vi "HMI_script_Generator.vi"(9 "Table Name":string, 10 "Columns":string[](array[string]), 11 "column information":T2(array[cluster])) -> (3 "HMI Script":string)   [LabVIEW 2020]
uses:
  <vilib>/addons/database/Auxilliary.llb/DB Tools DataTypes.ctl
  <userlib>/_OpenG.lib/array/array.llb/Search 1D Array (String)__ogtk.vi
  <userlib>/_OpenG.lib/array/array.llb/Delete Elements from 1D Array (String)__ogtk.vi
  <vilib>/regexp/Match Regular Expression.xnode
  <vilib>/addons/database/NI_Database_API.lvlib
panel:
  out "MACHINE NO":string
  out "Indices of Elements":i32[](array[numeric])
  out "column information 2":T2(array[cluster])
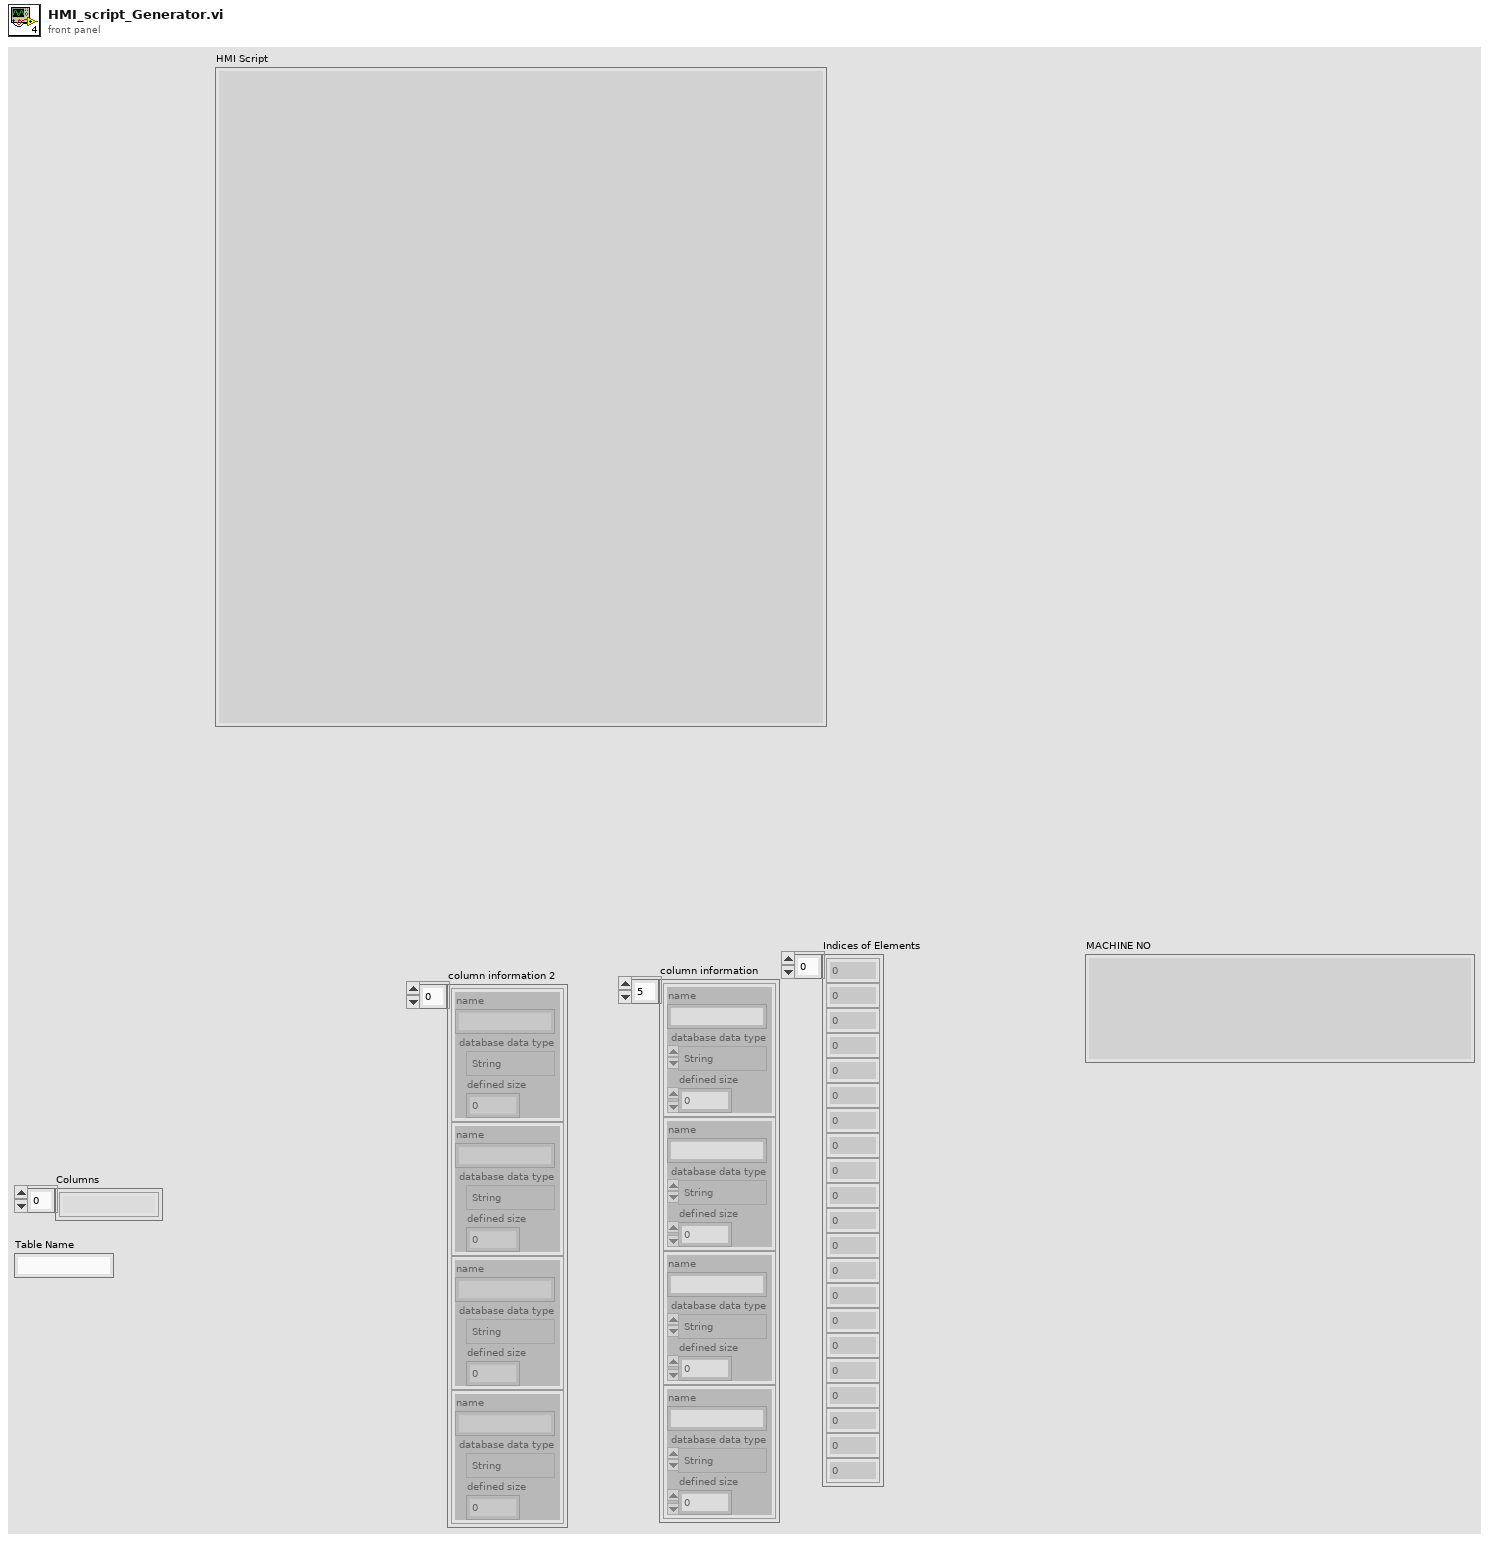
[diagram p1: front panel]
types:
  T1 = typedef "NI_Database_API.lvlib/DB Tools DataTypes.ctl" = enum16{"String", "Long (I32)", "Single (SGL)", "Double (DBL)", "Date/Time", "Binary"}
  T2 = cluster{"name":string, "database data type":T1, "defined size":i32}[]
  T3 = cluster{"name":string, "database data type":T1, "defined size":i32}
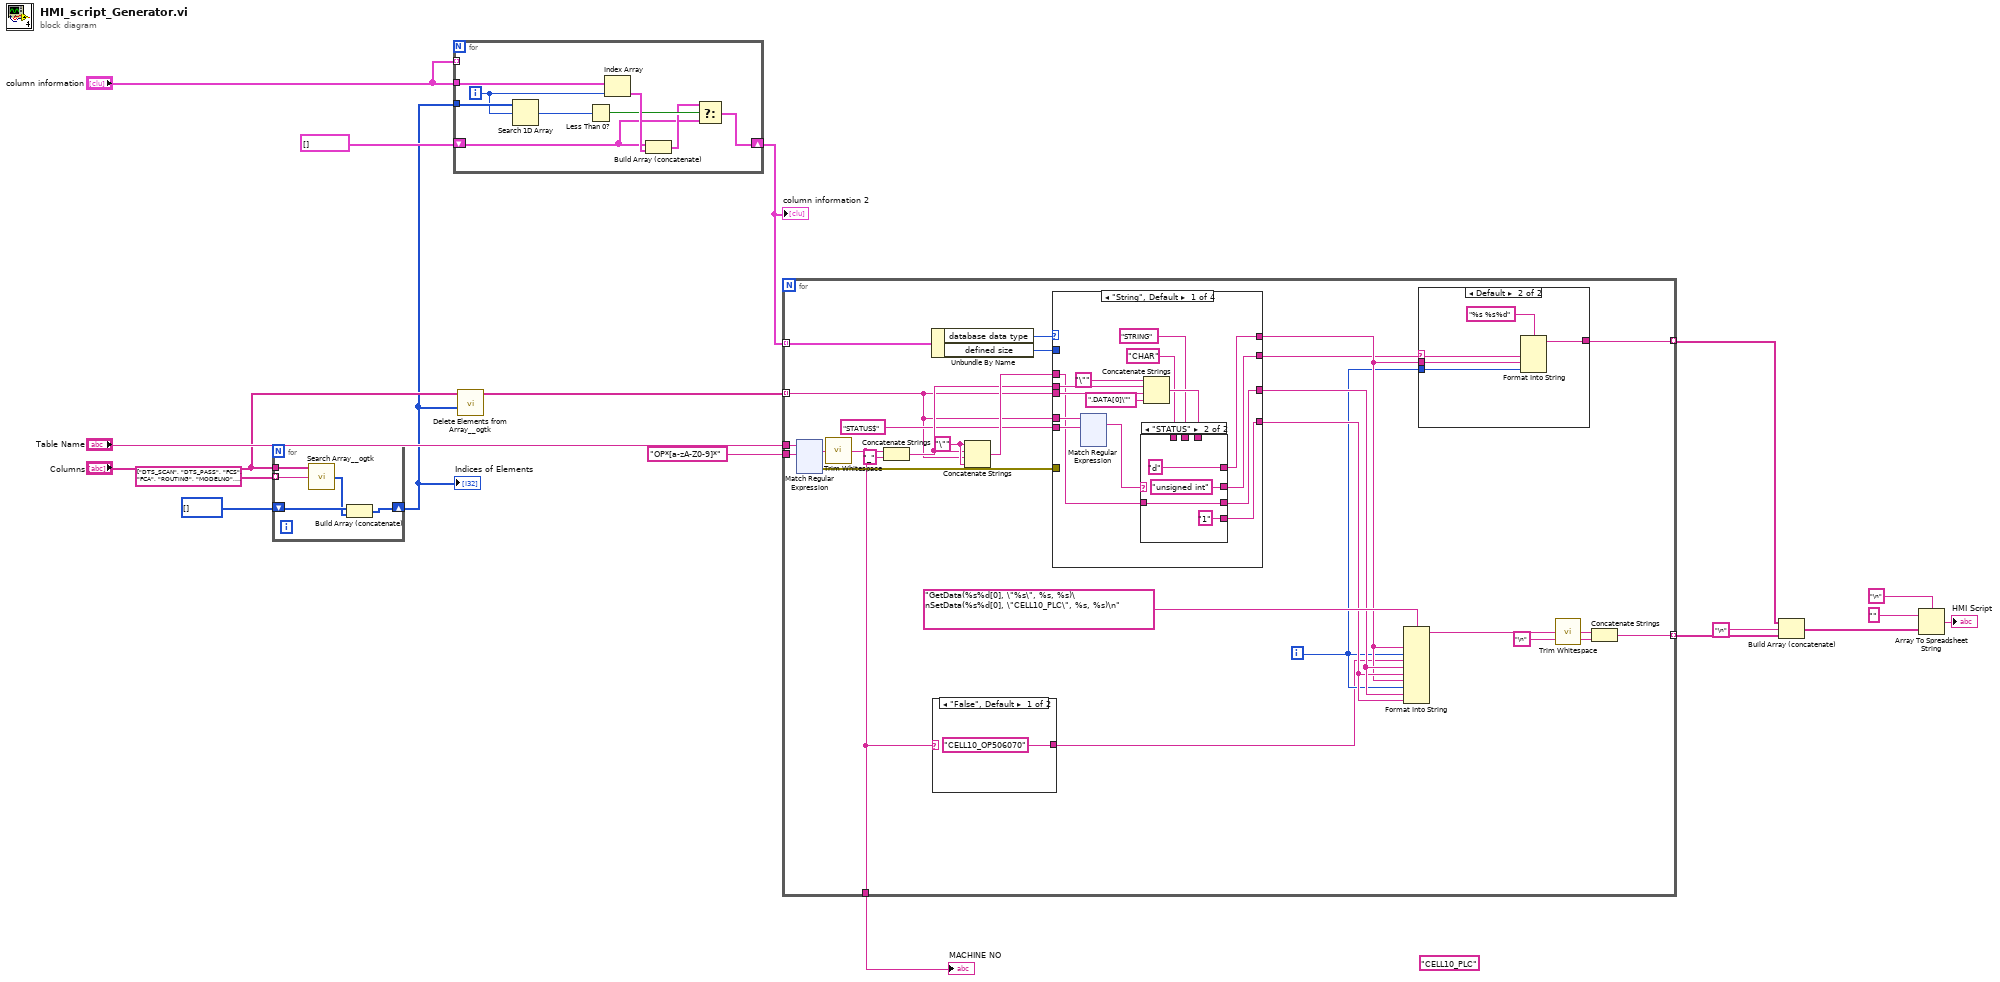
[diagram p0: block diagram]
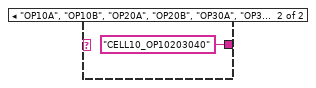
[diagram p2: hidden frame]
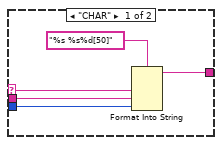
[diagram p3: hidden frame]
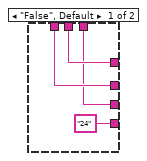
[diagram p4: hidden frame]
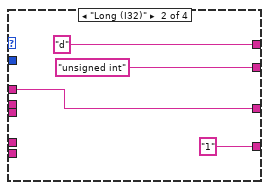
[diagram p5: hidden frame]
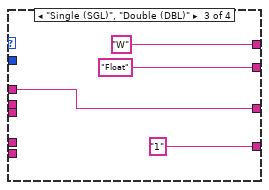
[diagram p6: hidden frame]
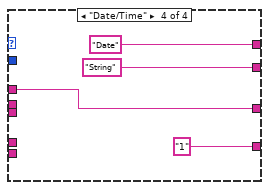
[diagram p7: hidden frame]
diagram:
  (unwired) "CELL10_PLC" ("format string")
  n1 = for {
    tunnel: "Columns" -> [w23]
    tunnel: string[] ["DTS_SCAN", "DTS_PASS", "FCS", "FCA", "ROUTING", "MODELNO", "WORKORDER", "CELLNO", "PROFITCENTRE", "MACHINECODE", "OPERATIONCODE"] ("columns") -> [w22] mode=indexing
    shift-right: [w20] -> w10
    shift-left: i32[] [] ("Indices of Elements") -> [w21]
    n2 = call-poly <userlib>:"Search Array__ogtk.vi"("Array"=w23, "Element Data"=w22) -> ("Indices of Elements"=w19:i32[])  [unwired: 7 in]
    n3 = Build Array (concatenate)(w21, w19) -> (w20:i32[])
  }
  "Indices of Elements" <- w10
  n4 = for {
    tunnel: "column information" -> [w32]
    shift-right: [w27] -> w14
    shift-left: T2 [] ("column information") -> [w28]
    tunnel: w10 -> [w26]
    tunnel: "column information" -> [_] mode=indexing
    i -> [w25]
    n5 = Search 1D Array(1D array=w26, element=w25) -> (index of element=w24:i32)  [unwired: 1 in]
    n6 = Less Than 0?(x=w24) -> (x < 0?=w30:bool)
    n7 = Index Array(array=w32, index=w25) -> (element=w31:T3)
    n8 = Build Array (concatenate)(w28, w31) -> (w29:T2)
    n9 = Select(t=w29, s=w30, f=w28) -> (s? t:f=w27:T2)
  }
  "column information 2" <- w14
  n10 = call-poly <userlib>:"Delete Elements from Array__ogtk.vi"("indices"=w10, "array"="Columns") -> ("array w/ subset deleted"=w12:string[])  [unwired: 8 in, 1 out]
  n11 = for {
    tunnel: w14 -> [w58] mode=indexing
    tunnel: "OP*[a-zA-Z0-9]*" ("String") -> [w56]
    tunnel: w12 -> [w35] mode=indexing
    tunnel: "Table Name" -> [w52]
    tunnel: [w34] -> w8
    tunnel: [w44] -> w7 mode=indexing
    tunnel: [w38] -> w2 mode=indexing
    i -> [w39]
    w50 = "\"" ("string")
    n12 = xnode "Match Regular Expression"("input string"=w52, "regular expression"=w56) -> ("whole match"=w53:string, "error out"=w51:errorcluster)  [unwired: 4 in, 3 out]
    n13 = call <vilib>:"Trim Whitespace.vi"("string"=w53) -> ("trimmed string"=w34:string)  [unwired: 1 in]
    n14 = Concatenate Strings(w34, "_" ("string")) -> (w48:string)
    n15 = Unbundle By Name(w58) -> ("database data type"=w55:T1, "defined size"=w57:i32)
    n16 = case shown="\"False\", Default" w34 {
      tunnel: ["CELL10_OP506070" ("format string") "CELL10_OP10203040" ("format string")] -> w33
      frame "False", Default {
      }
      frame "OP10A", "OP10B", "OP20A", "OP20B", "OP30A", "OP30B", "OP40A", "OP40B" {
      }
    }
    n17 = Concatenate Strings(w50, w48, w35, w50) -> (w54:string)
    n18 = case shown="\"String\", Default" w55 {
      tunnel: w57 -> [_ _ _ _]
      tunnel: w51 -> [_ _ _ _]
      tunnel: [w186 "d" "W" "Date"] -> w40
      tunnel: w54 -> [w192 w324 w328 w333]
      tunnel: w35 -> [w199 _ _ _]
      tunnel: [w190 w324 w328 w333] -> w42
      tunnel: w48 -> [w196 _ _ _]
      tunnel: [w185 "1" ("string") "1" ("string") "1" ("string")] -> w41
      tunnel: [w188 "unsigned int" "Float" "String"] -> w37
      tunnel: "STATUS$" -> [w194 _ _ _]
      tunnel: w35 -> [w193 _ _ _]
      frame "String", Default {
        n19 = xnode "Match Regular Expression"("input string"=w193, "regular expression"=w194) -> ("whole match"=w195:string)  [unwired: 4 in, 4 out]
        n20 = Concatenate Strings("\"" ("string"), w196, w199, ".DATA[0]\"" ("string")) -> (w191:string)
        n21 = case shown="\"STATUS\"" w195 {
          tunnel: [w316 "unsigned int"] -> w188
          tunnel: [w317 "d"] -> w186
          tunnel: "STRING" -> [w317 _]
          tunnel: "CHAR" -> [w316 _]
          tunnel: w191 -> [w315 _]
          tunnel: [w315 w319] -> w190
          tunnel: w192 -> [_ w319]
          tunnel: ["24" ("string") "1" ("string")] -> w185
          frame "False", Default {
          }
          frame "STATUS" {
          }
        }
      }
      frame "Long (I32)" {
      }
      frame "Single (SGL)", "Double (DBL)" {
      }
      frame "Date/Time" {
      }
    }
    n22 = Format Into String(format string="GetData(%s%d[0], \"%s\", %s, %s)\nSetData(%s%d[0], \"CELL10_PLC\", %s, %s)\n", w40, w39, w33, w42, w41, w40, w39, w42, w41) -> (resulting string=w46:string)  [unwired: 2 in, 1 out]
    n23 = case shown="Default" w37 {
      selector: w37 -> [w61 w66]
      tunnel: w40 -> [w64 w69]
      tunnel: w39 -> [w63 w68]
      tunnel: [w62 w67] -> w38
      frame "CHAR" {
        n24 = Format Into String(format string="%s %s%d[50]", w61, w64, w63) -> (resulting string=w62:string)  [unwired: 2 in, 1 out]
      }
      frame Default {
        n25 = Format Into String(format string="%s %s%d", w66, w69, w68) -> (resulting string=w67:string)  [unwired: 2 in, 1 out]
      }
    }
    n26 = call <vilib>:"Trim Whitespace.vi"("string"=w46) -> ("trimmed string"=w45:string)  [unwired: 1 in]
    n27 = Concatenate Strings(w45, "\n" ("string")) -> (w44:string)
  }
  "MACHINE NO" <- w8
  n28 = Build Array (concatenate)(w2, "\n" ("delimiter (Tab)"), w7) -> (w3:string[])
  n29 = Array To Spreadsheet String(delimiter (Tab)="\n", array=w3, 3:"" ("format string")) -> (spreadsheet string=→"HMI Script":string)
